vi "FTW-Endpoint-Destroy.vi"(0 "FTW Endpoint":refnum<class "FTW-Endpoint-Notifier.lvclass">, 5 "Force Destroy":bool, 11 "error in":errorcluster) -> (15 "error out":errorcluster)   [LabVIEW 2012, in "FTW-Actor.lvlib" / "FTW-Endpoint-Notifier.lvclass"]
uses:
  FTW-Endpoint-Notifier.lvclass
  FTW-Endpoint-Notifier.lvclass/FTW-Endpoint-Notifier.ctl
panel:
  # "Inputs"
  # "Outputs"
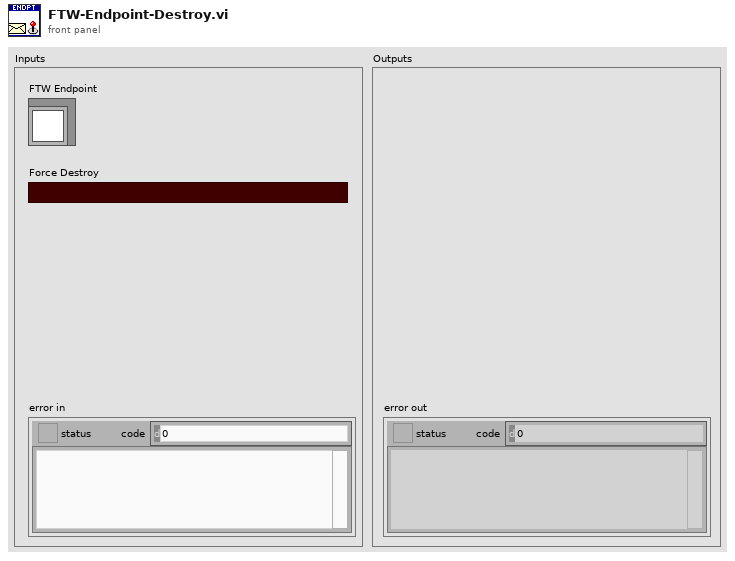
[diagram p1: front panel]
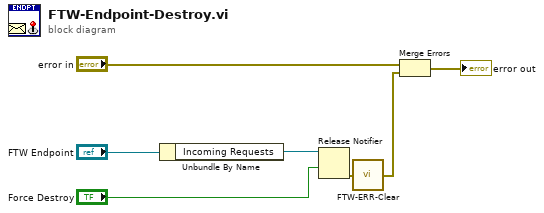
[diagram p0: block diagram]
diagram:
  n1 = Unbundle By Name("FTW Endpoint") -> ("Incoming Requests"=w6:refnum<notifier>)
  n2 = Release Notifier(notifier=w6, force destroy? (F)="Force Destroy") -> (error out=w2:errorcluster)  [unwired: 1 in, 2 out]
  n3 = call "FTW-ERR-Clear.vi"("error to snuff"=w2) -> ("no error"=w1:errorcluster)
  n4 = Merge Errors("error in", w1) -> (→"error out":errorcluster)
